vi "Add Instrument.vi"(8 "error in":errorcluster, 10 "Instrument":refnum<class "Instrument.lvclass">, 11 "MSS in":refnum<class "Measure and Stimulus Subsystems.lvclass">) -> (0 "error out":errorcluster, 3 "MSS out":refnum<class "Measure and Stimulus Subsystems.lvclass">)   [LabVIEW 2023, in "HAL GOOP4.lvlib" / "Measure and Stimulus Subsystems.lvclass"]
uses:
  Measure and Stimulus Subsystems.lvclass
  Instrument/Instrument.lvclass
  Measure and Stimulus Subsystems.lvclass/Measure and Stimulus Subsystems.ctl
  <vilib>/Utility/miscctls.llb/LVMapReplaceAction.ctl
  Instrument/utils/Instrument_GetAttributes.vi
  <vilib>/Utility/error.llb/Error Cluster From Error Code.vi
  <vilib>/ErrorRing/Error Ring.xnode
  Interfaces/IConfigure/IConfigure.lvclass
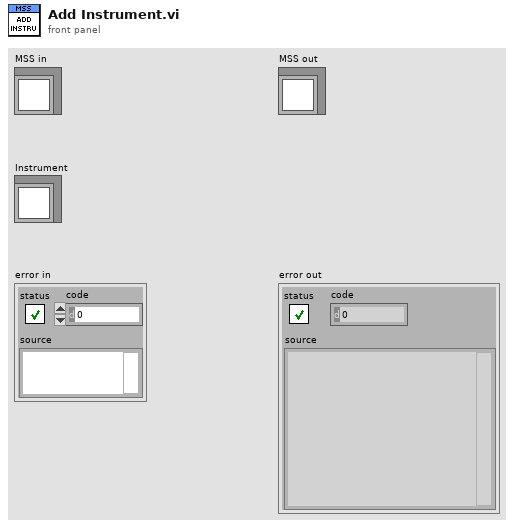
[diagram p1: front panel]
types:
  T1 = typedef "LVMapReplaceAction.ctl" = enum32{"Modify Entry only if found", "Add or Modify Entry", "Delete Entry"}
  T2 = map{string, cluster{"Instrument":refnum<class "Instrument.lvclass">, "Ref Count":u8}}
  T3 = cluster{"Instrument":refnum<class "Instrument.lvclass">, "Ref Count":u8}
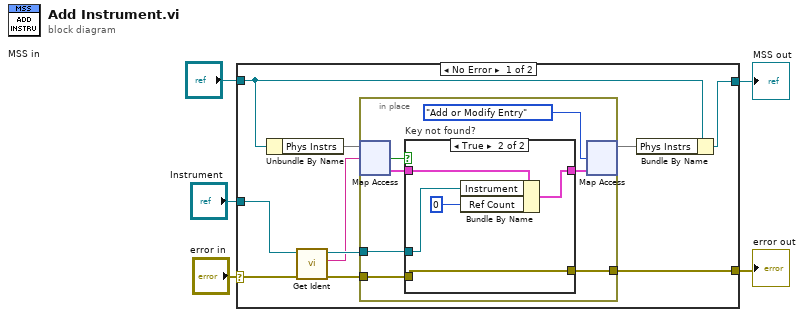
[diagram p0: block diagram]
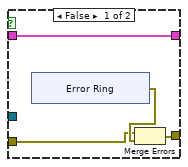
[diagram p2: hidden frame]
diagram:
  n1 = case shown="No Error" "error in" {
    selector: "error in" -> [w6 w38]
    tunnel: "Instrument" -> [w15 _]
    tunnel: "MSS in" -> [w9 w37]
    tunnel: [w8 w37] -> w3
    tunnel: [w7 w38] -> w2
    frame No Error {
      n2 = Unbundle By Name(w9) -> ("Phys Instrs"=w13:T2)
      n3 = call "Get Ident.vi"("Error In"=w6, "reference in"=w15) -> ("Error Out"=w10:errorcluster, "Instr Ident"=w11:string, "reference out"=w12:refnum<class "Instrument.lvclass">)  [unwired: 7 in]
      n4 = in-place {
        in-place-border: w12 -> [w20]
        in-place-border: w10 -> [w17]
        in-place-border: [w16] -> w7
        n5 = in-place-map #1(w13, w11) -> (w21:T3, w22:bool)  [unwired: 1 in]
        n6 = case "Key not found?" shown="True" w22 {
          tunnel: w21 -> [w23 w33]
          tunnel: [w23 w35] -> w18
          tunnel: w20 -> [_ w36]
          tunnel: w17 -> [w25 w34]
          tunnel: [w24 w34] -> w16
          frame False {
            n7 = xnode "Error Ring"() -> ("error out"=w26:errorcluster)
            n8 = Merge Errors(w25, w26) -> (w24:errorcluster)
          }
          frame True {
            n9 = Bundle By Name(cluster=w33, "Instrument"=w36, "Ref Count"=u8 0) -> (w35:T3)
          }
        }
        n10 = in-place-map #1(w18, LVMapReplaceAction."Add or Modify Entry" ("action")) -> (w14:T2)  [unwired: 2 out]
      }
      n11 = Bundle By Name(cluster=w9, "Phys Instrs"=w14) -> (w8:refnum<class "Measure and Stimulus Subsystems.lvclass">)
    }
    frame Error {
    }
  }
  "error out" <- w2
  "MSS out" <- w3
